vi "Flock_Logger_Log To File.vi"(8 "error in":errorcluster, 10 "Text":string, 11 "File":path=path "C:/FlockLog.txt") -> (0 "error out":errorcluster, 2 "TextOut":string)   [LabVIEW 2013, in "Logger.lvlib"]
doc: "Opens/Creates the log file and adds latest information."
uses:
  Logger.lvlib
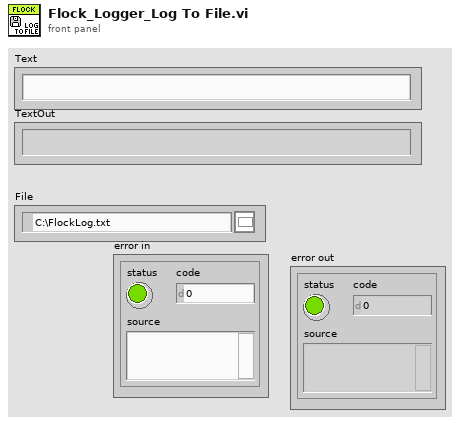
[diagram p1: front panel]
types:
  T1 = enum16{"open", "replace", "create", "open or create", "replace or create", "replace or create with confirmation"}
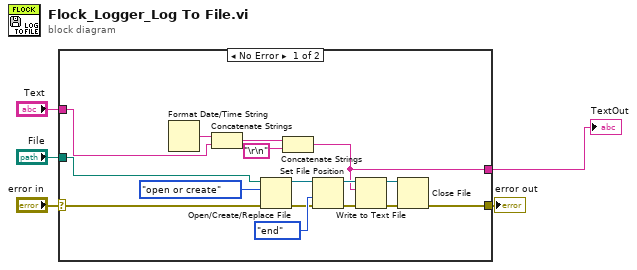
[diagram p0: block diagram]
diagram:
  n1 = case shown="No Error" "error in" {
    selector: "error in" -> [w21 w22]
    tunnel: [w20 w22] -> w5
    tunnel: "Text" -> [w8 _]
    tunnel: "File" -> [w7 _]
    tunnel: [w6 _] -> w1
    frame No Error {
      n2 = Format Date/Time String() -> (date/time string=w16:string)  [unwired: 3 in]
      n3 = Concatenate Strings(w16, w8) -> (w17:string)
      n4 = Open/Create/Replace File(file path (use dialog)=w7, error in=w21, operation (0:open)=T1."open or create") -> (refnum out=w15:refnum<file>, error out=w14:errorcluster)  [unwired: 3 in, 1 out]
      n5 = Concatenate Strings(w17, "\r\n") -> (w6:string)
      n6 = Set File Position(refnum=w15, from (0:start)=enum16{"start", "end", "current"}."end" ("pos mode (0:2)"), error in=w14) -> (refnum out=w13:refnum<file>, error out=w12:errorcluster)  [unwired: 1 in]
      n7 = Write to Text File(file (use dialog)=w13, text=w6, error in=w12) -> (refnum out=w9:refnum<file>, error out=w10:errorcluster)  [unwired: 1 in, 1 out]
      n8 = Close File(refnum=w9, error in=w10) -> (error out=w20:errorcluster)  [unwired: 1 out]
    }
    frame Error {
    }
  }
  "error out" <- w5
  "TextOut" <- w1
